vi "function generator.vi"(5 "Tx":dbl=0.5, 6 "ratio of decline":dbl=0.3, 7 "t_bgn":dbl=155706.6935322797, 8 "Row_N":i32=10, 9 "Vy_max":dbl=1.0, 10 "Vx_max":dbl=1.0, 11 "t_cur":dbl=155711.71098783312) -> (1 "finished?":i32, 2 "y":dbl, 3 "x":dbl)   [LabVIEW 2013]
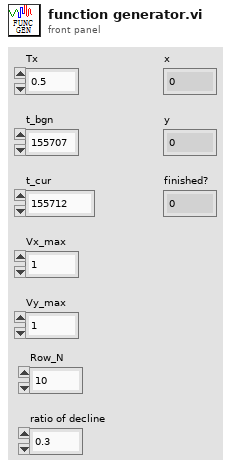
[diagram p1: front panel]
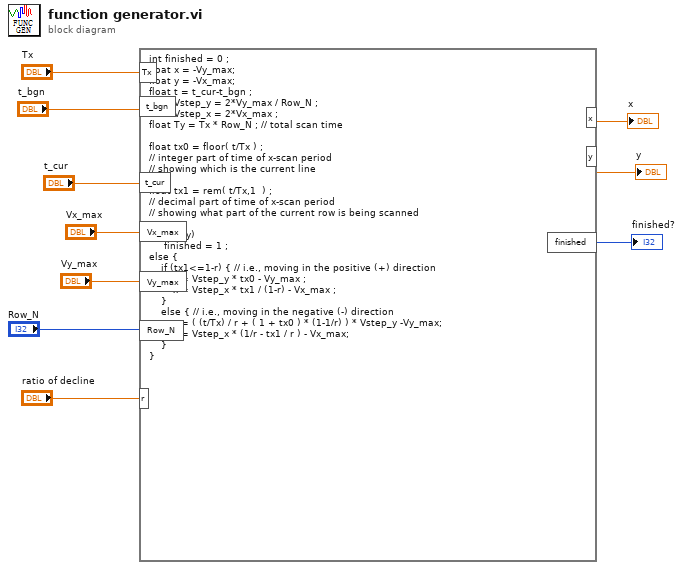
[diagram p0: block diagram]
diagram:
  n1 = formula code="int finished = 0 ;\nfloat x = -Vy_max;\nfloat y = -Vx_max;\nfloat t = t_cur-t_bgn ;\nfloat Vstep_y = 2*Vy_max / Row_N ;\nfloat Vstep_x = 2*Vx_max ;\nfloat Ty = Tx * Row_N ; // total scan time\n\nfloat tx0 = floor( t/Tx ) ;\n// integer part of time of x-scan period\n// showing which is the current line\n\nfloat tx1 = rem( t/Tx,1  ) ;\n// decimal part of time of x-scan period\n// showing what part of the current row is being scanned\n\nif (t > Ty)\n     finished = 1 ;\nelse {\n    if (tx1<=1-r) { // i.e., moving in the positive (+) direction\n        y = Vstep_y * tx0 - Vy_max ;\n        x = Vstep_x * tx1 / (1-r) - Vx_max ;\n    }\n    else { // i.e., moving in the negative (-) direction\n        y = ( (t/Tx) / r + ( 1 + tx0 ) * (1-1/r) ) * Vstep_y -Vy_max;\n        x = Vstep_x * (1/r - tx1 / r ) - Vx_max;\n    }\n}"("t_cur"="t_cur", "Vx_max"="Vx_max", "Vy_max"="Vy_max", "Row_N"="Row_N", "Tx"="Tx", "r"="ratio of decline", "t_bgn"="t_bgn") -> ("x"=→"x":dbl, "y"=→"y":dbl, "finished"=→"finished?":i32)
